vi "test_fpga_se_main_sid.vi"() -> ()   [LabVIEW 2016]
uses:
  <vilib>/Platform/TimedLoop/XDataNode/timing_clust.ctl
  <vilib>/Platform/TimedLoop/XDataNode/nitl_modes.ctl
  <vilib>/Platform/TimedLoop/XDataNode/wakeup.ctl
  <vilib>/rvi/Emulation/niFpgaSctlEmulationGetInTimedLoop.vi
  <vilib>/rvi/Emulation/niFpgaEmulationIsFPGAContextNoSignature.vi
  <vilib>/rvi/errors/niFpgaSetErrorForExecOnDevCompSimple.vi
  <vilib>/rvi/eio/common/nirviEmuReportErrorAndStop.vi
  <vilib>/rvi/DataTransferAndStorage/Container/Common/niFpgaContainerGetUniqueNameForEmu.vi
  <vilib>/rvi/FIFO/Fifo_Resource/nirvififoEmulationSetSize.vi
  <vilib>/rvi/FIFO/Fifo_Resource/nirviFifoEmulationQueueMgr.vi
  <instcachedir>/0/nirviFifoEmulationQueueMgr_E5CAEC123FF24DC58D834DCA3CDAA9B5.lvgen/nirviFifoEmulationQueueMgr_E5CAEC123FF24DC58D834DCA3CDAA9B5_012.vi
  <vilib>/rvi/FIFO/Fifo_Resource/nirvififoEmulationDetermineInputValidOut.vi
  <vilib>/rvi/FIFO/Fifo_Resource/nirvififoEmulationCreateLock.vi
  <vilib>/rvi/Emulation/niFpgaProcessEmulError.vi
  <vilib>/rvi/FIFO/Fifo_Resource/nirvififoEmulationObtainLock.vi
  <vilib>/rvi/FIFO/Fifo_Resource/nirvififoEmulationReleaseLock.vi
  <vilib>/rvi/occurrence/nirviWaitOnOccurrenceBase.vi
  <vilib>/rvi/errors/nirviReportUnexpectedCaseInternalError.vi
  <vilib>/rvi/errors/nirviReportUnexpectedCaseInternalError (U32).vi
  <vilib>/rvi/Memory/Memory_Emulation/nirvimemoryFastEmulation.vi
  <vilib>/rvi/Memory/Memory_Emulation/nirvimemoryEmulation.vi
  <vilib>/Platform/TimedLoop/XDataNode/XDataNode.xnode
  <vilib>/rvi/FXPMathLib/FxpInterpret/XNode/nifxpmath_Interpret.xnode
  <vilib>/rvi/DataTransferAndStorage/Container/XNode/niFpgaContainer.xnode
  <vilib>/rvi/FIFO/Fifo_Resource/nirvififoEmulationWrite.vi
  <vilib>/Platform/TimedLoop/XDataNode/XDNodeRunTimeDep.lvlib
panel:
  out "se.sid.itcOutput":bool
  out "se.sid.s.running":bool
  out "se.sid.s.repetitions":u16
  in  "se.sid.p.params":T1={"sysIdOutputRate"=100, "sysIdWaveSize"=4092, "sysIdRepetitions"=50, "high"=0.0, "low"=0.0} {"sysIdOutputRate" min=10}
  in  "se.sid.p.axisXNotY":bool=TRUE
  in  "se.sid.start":bool
  in  "se.sid.m.sequence":cluster{"write":bool, "data":bool, "index":u16}
  out "se.o.positionSID":T2 {"outputInt"."x" format="%.17g"; "outputInt"."y" format="%.17g"}
  in  "se.p.scanOffsets":cluster{"x":fxp<+/-,16,1>, "y":fxp<+/-,16,1>}
  in  "se.mot.p.target":cluster{"x":fxp<+/-,16,1>, "y":fxp<+/-,16,1>}
  out "se.mot.s.running":bool
  in  "se.p.transformMatrix":T3
  in  "se.p.scanSize":T4
  in  "se.p.clocks":T5={"outputRate"=50, "fastDecFactor"=0, "outWaveSizeFast"=0, "pplUpsampling"=0, "numLines"=0, "se.p.fastInvDec"=0.0, "se.p.slowUpStep"=0.0, "se.p.outWaveSizeSlow"=0, "blankingMax"=10000000, "se.p.fastBlanking"={"startFwd"=0, "endFwd"=10000, "startBwd"=0, "endBwd"=0, "disableBlanking"=FALSE, "useCoarseCounter"=TRUE}}
  in  "se.mot.p.clocks":T6
  out "se.mot.s.origin":T7
  in  "se.p.modes":T8
  out "se.s.blankingOff":bool
  out "se.o.position":T9 {"outputInt"."x" format="%.16g"; "outputInt"."y" format="%.16g"}
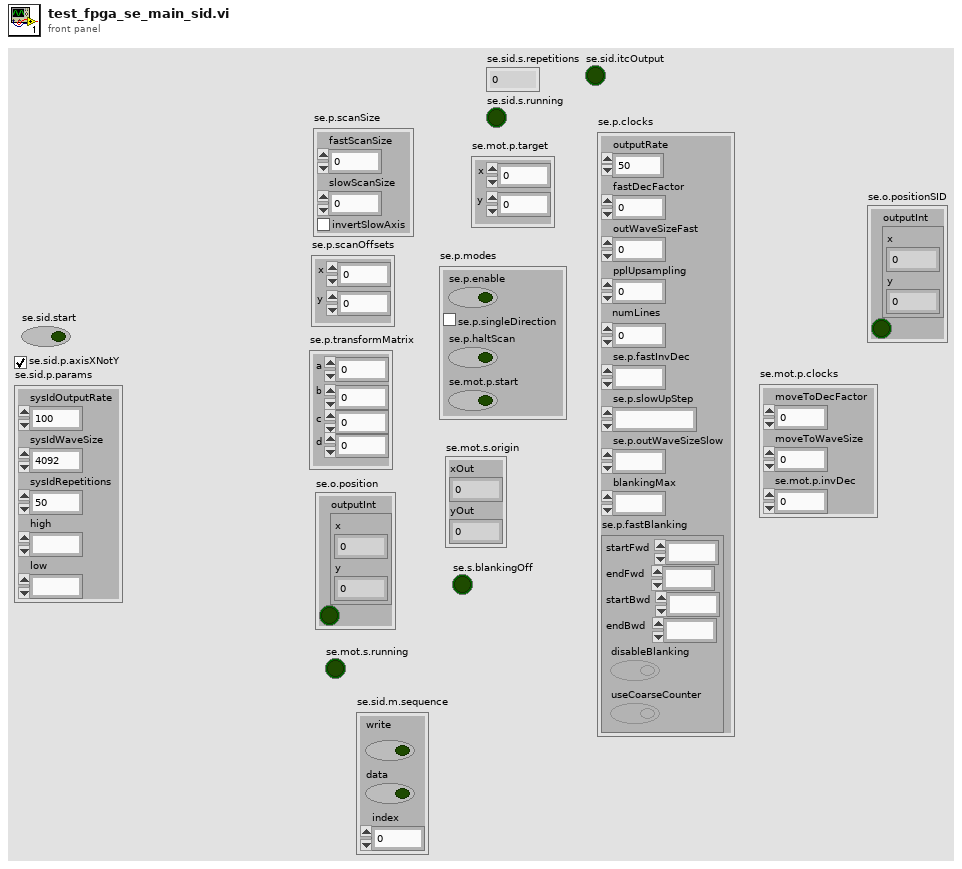
[diagram p1: front panel]
types:
  T1 = cluster{"sysIdOutputRate":u16, "sysIdWaveSize":u16, "sysIdRepetitions":u16, "high":fxp<+/-,17,1>, "low":fxp<+/-,17,1>}
  T2 = cluster{"outputInt":cluster{"sid.o.height":fxp<+/-,28,1>, "sid.o.height":fxp<+/-,28,1>}, bool}
  T3 = cluster{"a":fxp<+/-,18,2>, "b":fxp<+/-,18,2>, "c":fxp<+/-,18,2>, "d":fxp<+/-,18,2>}
  T4 = cluster{"fastScanSize":fxp<+,17,1>, "slowScanSize":fxp<+,17,1>, "invertSlowAxis":bool}
  T5 = cluster{"outputRate":u16, "fastDecFactor":u16, "outWaveSizeFast":u16, "pplUpsampling":u16, "numLines":u16, "se.p.fastInvDec":fxp<+,22,0>, "se.p.slowUpStep":fxp<+,28,0>, "se.p.outWaveSizeSlow":u16, "blankingMax":u32, "se.p.fastBlanking":cluster{"startFwd":u32, "endFwd":u32, "startBwd":u32, "endBwd":u32, "disableBlanking":bool, "useCoarseCounter":bool}}
  T6 = cluster{"moveToDecFactor":u16, "moveToWaveSize":u16, "se.mot.p.invDec":fxp<+,16,0>}
  T7 = cluster{"xOut":fxp<+/-,18,2>, "yOut":fxp<+/-,18,2>}
  T8 = cluster{"se.p.enable":bool, "se.p.singleDirection":bool, "se.p.haltScan":bool, "se.mot.p.start":bool}
  T9 = cluster{"outputInt":cluster{"y":fxp<+/-,16,1>, "y":fxp<+/-,16,1>}, bool}
  T10 = typedef "XDNodeRunTimeDep.lvlib/timing_clust.ctl" = cluster{"Expected End [f-1]":u64, "Actual End [f-1]":u64, "Finished Late? [f-1]":bool, "Expected End [i-1]":u64, "Actual End [i-1]":u64, "Finished Late? [i-1]":bool, "Expected Start [i]":u64, "Actual Start [i]":u64, "Expected Start [f]":u64, "Actual Start [f]":u64, "Source Name":string, "Structure Name":string, "Period":i64, "Deadline":i64, "Offset":i64, "Start":i64, "Priority":i32, "Timeout":i32, "Mode":T11, "Wakeup Reason":T12, "Error":errorcluster, "Source Type":string, "Secondary Source Type":string, "Global End Time":u64, "Global Start Time":u64, "Frame Duration":u64, "Iteration Duration":u64, "Assigned CPU":i32, "I/O Scan Engine Mode":u32}
  T11 = typedef "XDNodeRunTimeDep.lvlib/nitl_modes.ctl" = enum32{"No Change", "Process missed periods, maintain original phase", "Discard missed periods, maintain original phase", "Process missed periods, ignore original phase", "Discard missed periods, ignore original phase"}
  T12 = typedef "XDNodeRunTimeDep.lvlib/wakeup.ctl" = enum32{"Normal", "Aborted", "Asynchronous wakeup", "Timing source error", "Timed loop error", "Timeout"}
  T13 = cluster{"se.mot.p.clocks":cluster{"moveToDecFactor":u16, "moveToWaveSize":u16, "se.mot.p.invDec":fxp<+,16,0>}, "se.p.clocks":cluster{"outputRate":u16, "fastDecFactor":u16, "outWaveSizeFast":u16, "pplUpsampling":u16, "numLines":u16, "se.p.fastInvDec":fxp<+,22,0>, "se.p.slowUpStep":fxp<+,28,0>, "se.p.outWaveSizeSlow":u16, "blankingMax":u32, "se.p.fastBlanking":cluster{"startFwd":u32, "endFwd":u32, "startBwd":u32, "endBwd":u32, "disableBlanking":bool, "useCoarseCounter":bool}}}
  T14 = cluster{"se.p.scanOffsets":cluster{"x":fxp<+/-,16,1>, "y":fxp<+/-,16,1>}, "se.p.transformMatrix":cluster{"a":fxp<+/-,18,2>, "b":fxp<+/-,18,2>, "c":fxp<+/-,18,2>, "d":fxp<+/-,18,2>}, "se.p.scanSize":cluster{"fastScanSize":fxp<+,17,1>, "slowScanSize":fxp<+,17,1>, "invertSlowAxis":bool}}
  T15 = cluster{"x+y":fxp<+/-,18,2>, "x+y":fxp<+/-,18,2>}
  T16 = cluster{"sid.o.height":fxp<+/-,28,1>, "sid.o.height":fxp<+/-,28,1>}
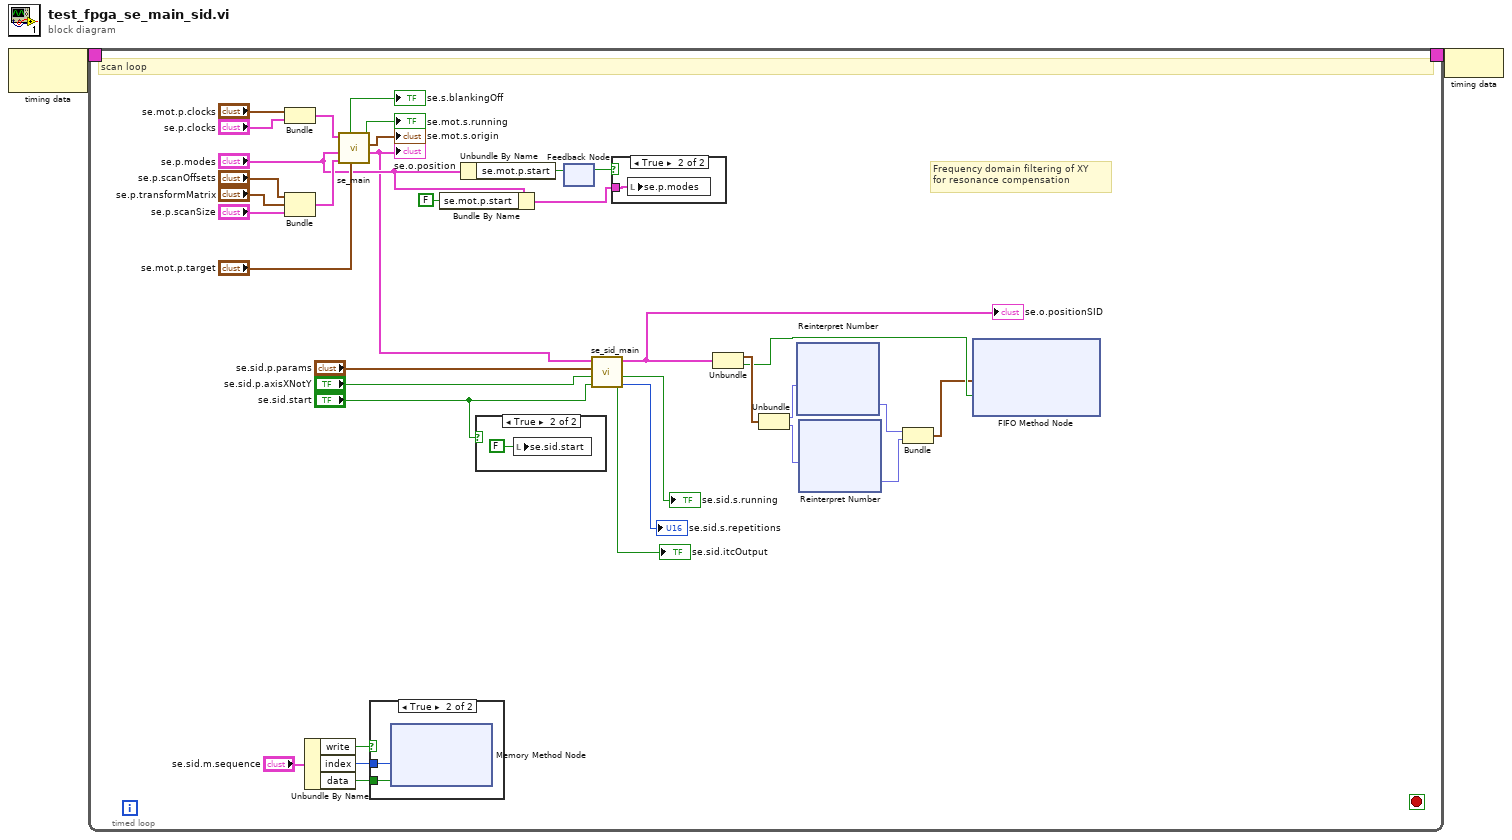
[diagram p0: block diagram]
diagram:
  n1 = node-c288() -> (w2:T10)  [unwired: 1 in]
  n2 = timed-loop {
    timing: w2 -> [_]
    timing-out: [_] -> w1
    stop <- _ stop-if-true
    # "Frequency domain filtering of XY \nfor resonance compensation"
    # "scan loop"
    n3 = Bundle("se.mot.p.clocks"="se.mot.p.clocks", "se.p.clocks"="se.p.clocks") -> (w30:T13)  [unwired: 1 in]
    n4 = Bundle("se.p.scanOffsets"="se.p.scanOffsets", "se.p.transformMatrix"="se.p.transformMatrix", "se.p.scanSize"="se.p.scanSize") -> (w29:T14)  [unwired: 1 in]
    n5 = Unbundle By Name("se.sid.m.sequence") -> ("write"=w19:bool, "index"=w20:u16, "data"=w21:bool)
    n6 = call "se_main.vi"("se.mot.p.target"="se.mot.p.target", "outputParams"=w29, "se.p.modes"="se.p.modes", "scanClocks"=w30) -> ("se.o.position"=w8:T9, "se.mot.s.origin"=→"se.mot.s.origin":T15, "se.mot.s.running"=→"se.mot.s.running":bool, "blankingOff"=→"se.s.blankingOff":bool)  [unwired: 1 in, 3 out]
    "se.o.position" <- w8
    n7 = case shown="True" w19 {
      tunnel: w20 -> [_ w40]
      tunnel: w21 -> [_ w39]
      frame False {
      }
      frame True {
        n8 = xnode ("Memory Method Node")("Address"=w40, "Data"=w39) -> ()  [unwired: 1 in, 1 out]
      }
    }
    n9 = Bundle By Name(cluster="se.p.modes", "se.mot.p.start"=FALSE) -> (w22:T8)
    n10 = Unbundle By Name("se.p.modes") -> ("se.mot.p.start"=w27:bool)
    n11 = case shown="True" "se.sid.start" {
      frame False {
      }
      frame True {
        n12 = local write "se.sid.start"(FALSE ("se.sid.start")) -> ()
      }
    }
    n13 = feedback-in #1(w27) -> ()
    n14 = feedback #1() -> (w23:bool)  [unwired: 1 in]
    n15 = call "se_sid_main.vi"("se.sid.start"="se.sid.start", "axisXNotY"="se.sid.p.axisXNotY", "sysIdParams"="se.sid.p.params", "se.sid.i.position"=w8) -> ("se.sid.s.repetitions"=→"se.sid.s.repetitions":u16, "se.sid.s.running"=→"se.sid.s.running":bool, "se.sid.o.position"=w9:T2, "se.sid.itcOutput"=→"se.sid.itcOutput":bool)  [unwired: 4 in]
    "se.o.positionSID" <- w9
    n16 = case shown="True" w23 {
      tunnel: w22 -> [_ w41]
      frame False {
      }
      frame True {
        n17 = local write "se.p.modes"(w41) -> ()
      }
    }
    n18 = Unbundle(w9) -> ("outputInt"=w13:T16, w7:bool)
    n19 = Unbundle(w13) -> ("sid.o.height"=w15:fxp<+/-,28,1>, "sid.o.height"=w16:fxp<+/-,28,1>)
    n20 = xnode "Reinterpret Number"("x"=w15) -> ("y"=w14:fxp<+/-,28,16>)
    n21 = xnode "Reinterpret Number"("x"=w16) -> ("y"=w17:fxp<+/-,28,16>)
    n22 = Bundle("y"=w14, "y"=w17) -> (w6:cluster{"y":fxp<+/-,28,16>, "y":fxp<+/-,28,16>})  [unwired: 1 in]
    n23 = xnode ("FIFO Method Node")("Element"=w6, "Input Valid"=w7) -> ()  [unwired: 1 in, 2 out]
  }
  n24 = node-c288(w1) -> ()
